vi "DaxsonicsGUI_3Pulsers.vi"(0 "Daxsonics VISA":refnum<visa-resource-name>="COM8", 5 "Daxsonics Name":T1, 11 "Uniform Gain":bool=TRUE) -> ()   [LabVIEW 2022 SP3]
doc: "This application VI allows the user to set the desired parameters in the Daxsonics BP2"
uses:
  -DaxSubroutines/Daxsonics_Pulsers.ctl
  PulserGlobals.vi
panel:
  in  "+12 dB Gain":bool
  in  "Element":u16(ring) items=["1", "2", "3", "4", "5"]
  in  "Delay Table (ns)":i32[][](array[numeric])=[[0, -1, -1, -1, -1], [-1, 0, -1, -1, -1], [-1, -1, 0, -1, -1], [-1, -1, -1, 0, -1], [-1, -1, -1, -1, 0]]
  in  "PRI":i32=500000
  in  "Trigger Rising (T)/Falling (F)":bool=TRUE
  in  "Trigger Ext(T)/Int(F)":bool
  in  "Freq (MHz)":u16(ring)=20 items=["50"=20, "45"=27, "40"=34, "35"=41, "30"=49, "25"=56, "20"=63, "15"=70]
  in  "Voltage (V)":u16(ring) items=["100"=100, "90"=90, "80"=80, "70"=70, "60"=60, "50"=50, "40"=40, "30"=30, "20"=20, "10"=10, "0"=0]
  in  "Gains (dB)":u16[](array[ring]) items=["64"=64, "60"=60, "52"=52, "48"=48, "44"=44, "40"=40, "36"=36, "32"=32, "28"=28, "24"=24, "20"=20, "16"=16]
  in  "Lock/Unlock":bool
  in  "ExitSendCmd":bool
  # "ONLY USED FOR 2021 NEW VERSION"
  # "Fixed 15.5 dB is start Gain"
  # "NUMTX = Rows\nColumn = Delays\n-1 means not used"
  # "Select xmit element (ie row)"
  # "Need to change COM port to these aliases based on daxsonics that is used\n\nDax2021 - newest Daxsonics from 2021\n\nor unites based on serial #\nDaxsonics_BP1 (faulty out of use)\nDaxsonics_BP2_A\nDaxsonics_BP2_B\n10ERS8 (this one is dead)"
  # "This is set up to pass one row"
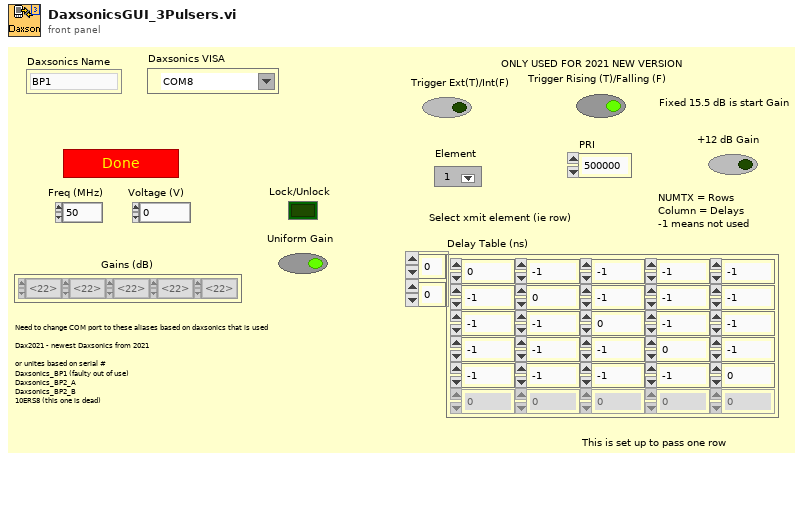
[diagram p1: front panel]
types:
  T1 = typedef "Daxsonics_Pulsers.ctl" = enum16{"BP1", "BP2_A", "BP2_B", "10ERS8", "New2021"}
  T2 = typedef "LVStringsAndValuesArrayTypeDef_U16.ctl" = cluster{"String":string, "Value":u16}[]
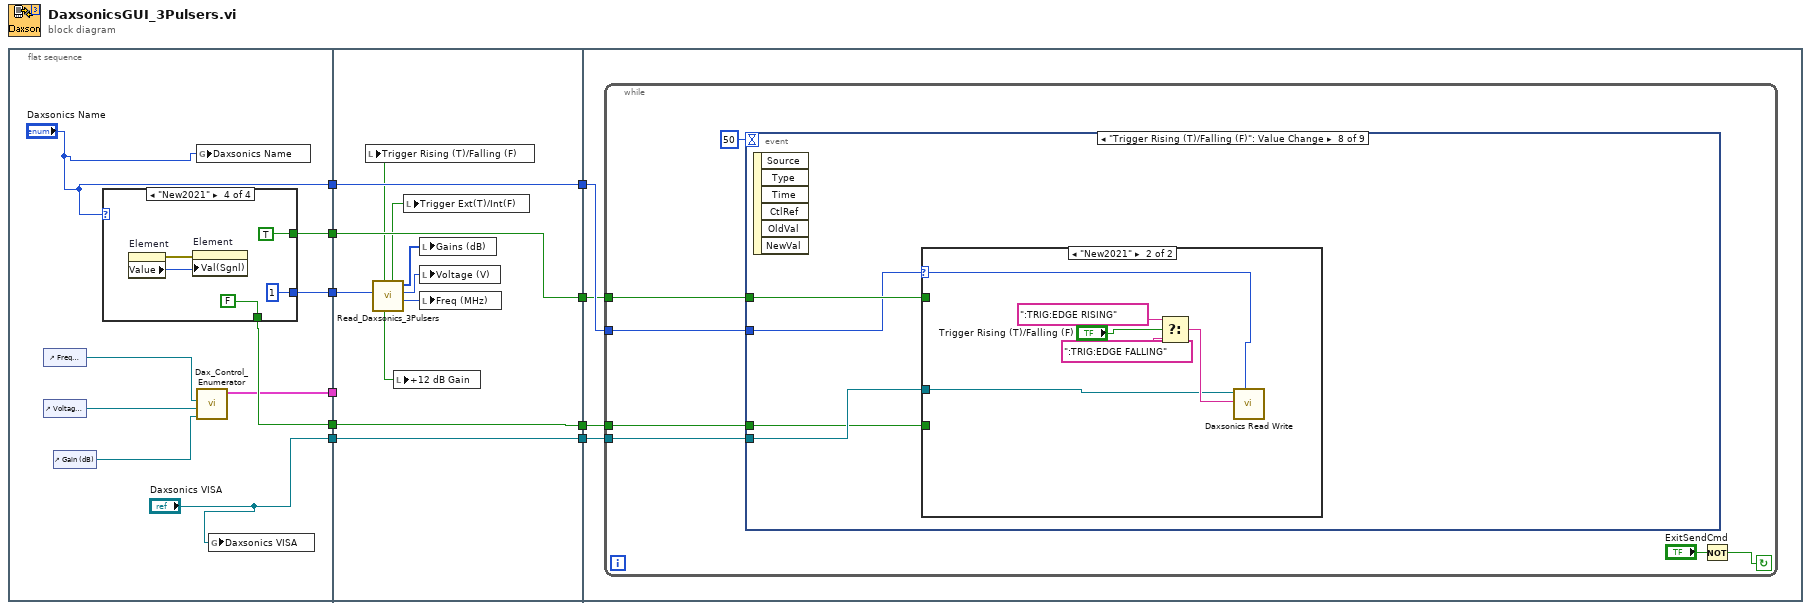
[diagram p0: block diagram]
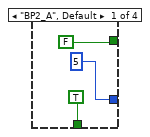
[diagram p2: hidden frame]
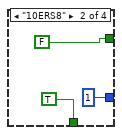
[diagram p3: hidden frame]
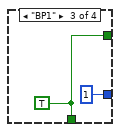
[diagram p4: hidden frame]
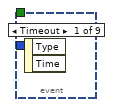
[diagram p5: hidden frame]
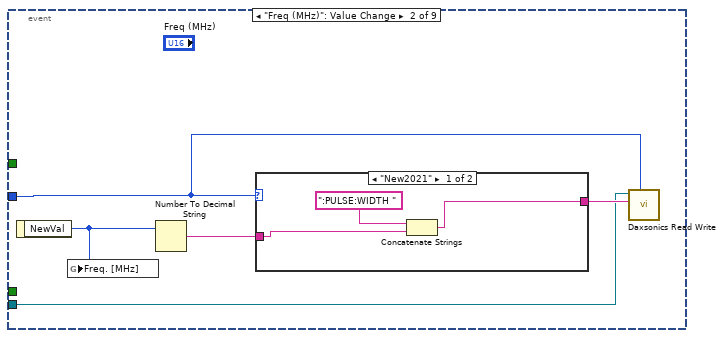
[diagram p6: hidden frame]
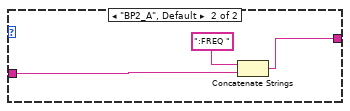
[diagram p7: hidden frame]
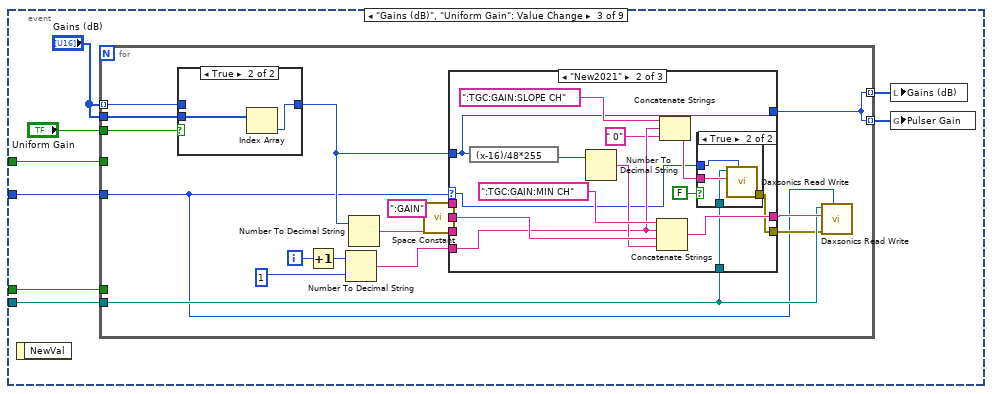
[diagram p8: hidden frame]
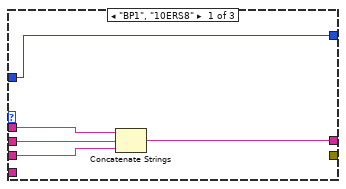
[diagram p9: hidden frame]
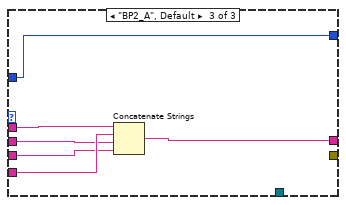
[diagram p11: hidden frame]
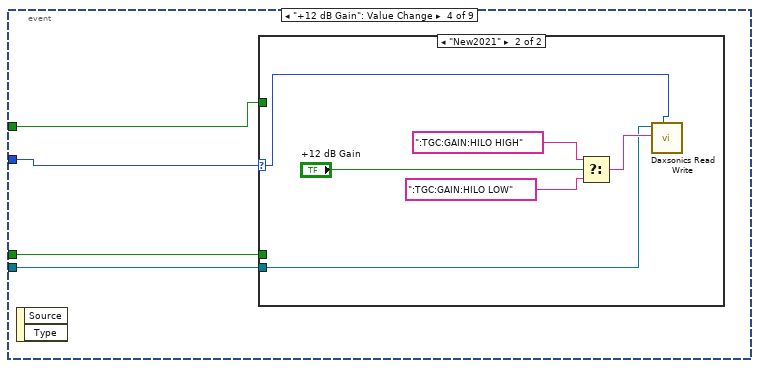
[diagram p13: hidden frame]
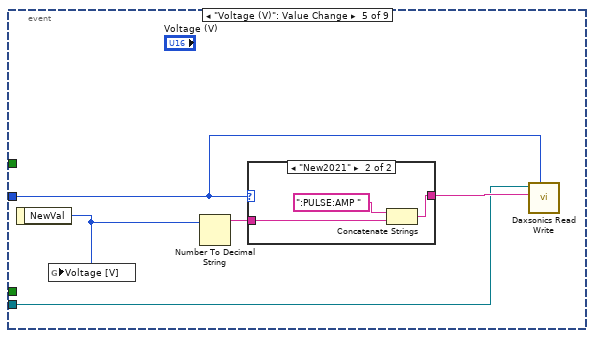
[diagram p15: hidden frame]
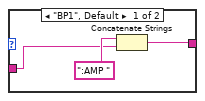
[diagram p16: hidden frame]
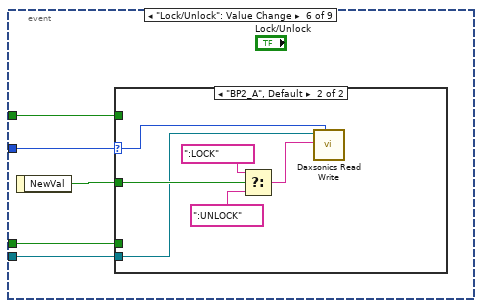
[diagram p17: hidden frame]
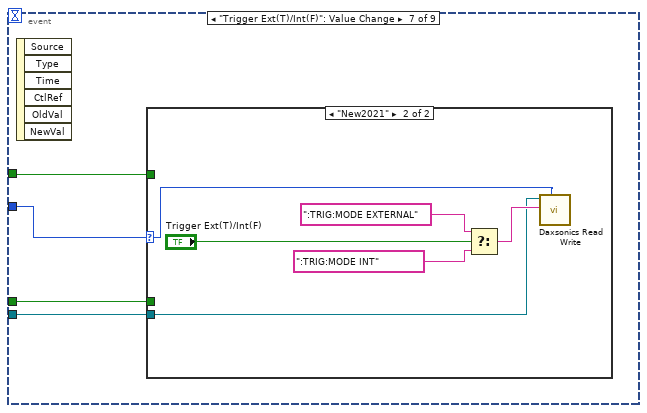
[diagram p19: hidden frame]
diagram:
  n1 = flat-sequence {
    tunnel: [w19] -> w9
    tunnel: ["Daxsonics Name"] -> w8
    tunnel: [w17] -> w5
    tunnel: [w14] -> w4
    tunnel: ["Daxsonics VISA"] -> w2
    tunnel: [w11] -> w1
    tunnel: [w33] -> w10
    tunnel: w9 -> [w40]
    tunnel: w8 -> [w39]
    tunnel: [w39] -> w7
    tunnel: [w38] -> w6
    tunnel: w5 -> [w38]
    tunnel: w4 -> [w37]
    tunnel: [w37] -> w3
    tunnel: w2 -> [w33]
    tunnel: w1 -> [_]
    tunnel: w10 -> [w47]
    tunnel: w7 -> [w46]
    tunnel: w6 -> [w45]
    tunnel: w3 -> [w44]
    frame #0 {
      n2 = control-ref of="Freq (MHz)"() -> (w18:refnum<vi>)
      n3 = control-ref of="Voltage (V)"() -> (w15:refnum<vi>)
      n4 = control-ref of="Gain (dB)"() -> (w16:refnum<vi>)
      n5 = case shown="\"New2021\"" "Daxsonics Name" {
        tunnel: [5 ("Num Channels") 1 ("Num Channels") 1 ("Num Channels") 1 ("Num Channels")] -> w19
        tunnel: [FALSE ("Enable Termination\nChar (T)") FALSE ("Enable Termination\nChar (T)") w26 TRUE ("Enable Termination\nChar (T)")] -> w17
        tunnel: [TRUE ("Enable Termination\nChar (T)") TRUE ("Enable Termination\nChar (T)") w26 FALSE ("Enable Termination\nChar (T)")] -> w14
        frame "BP2_A", Default {
        }
        frame "10ERS8" {
        }
        frame "BP1" {
          w26 = TRUE ("Enable Termination\nChar (T)")
        }
        frame "New2021" {
          n6 = property on="Element" class="Ring (strict)"() -> (error out=w29:errorcluster, "Value"=w28:u16)  [unwired: 2 in, 1 out]
          n7 = property on="Element" class="Ring (strict)"(error in=w29, "Val(Sgnl)"=w28) -> ()  [unwired: 1 in, 2 out]
        }
      }
      n8 = global write "PulserGlobals.vi" "Daxsonics Name"("Daxsonics Name") -> ()
      n9 = call "Dax_Control_Enumerator.vi"("Gain (dB) Ref"=w16, "Voltage (V) Ref"=w15, "Freq (MHz) Ref"=w18) -> ("Freq"=w11:T2)  [unwired: 6 in, 2 out]
      n10 = global write "PulserGlobals.vi" "Daxsonics VISA"("Daxsonics VISA") -> ()
    }
    frame #1 {
      n11 = call "Read_Daxsonics_3Pulsers.vi"("Num Channels"=w40) -> ("Freq (MHz)"=w43:u16, "Voltage (V)"=w42:u16, "Gains"=w41:u16[], "Trigger Ext(T)/Int(F)"=w35:bool, "HI(T)/LO(F) +12 dB"=w34:bool, "Trigger Rising (T)/Falling (F)"=w36:bool)  [unwired: 4 in, 1 out]
      n12 = local write "Trigger Rising (T)/Falling (F)"(w36) -> ()
      n13 = local write "+12 dB Gain"(w34) -> ()
      n14 = local write "Trigger Ext(T)/Int(F)"(w35) -> ()
      n15 = local write "Gains (dB)"(w41) -> ()
      n16 = local write "Voltage (V)"(w42) -> ()
      n17 = local write "Freq (MHz)"(w43) -> ()
    }
    frame #2 {
      n18 = while {
        tunnel: w47 -> [w51]
        tunnel: w46 -> [w50]
        tunnel: w45 -> [w49]
        tunnel: w44 -> [w48]
        stop <- w54 continue-if-true
        n19 = event shown="[7] \"Trigger Rising (T)/Falling (F)\": Value Change" {
          selector: _ -> [_ _ _ _ _ _ _ _ _]
          dyn-events: _ -> [_ _ _ _ _ _ _ _ _]
          timeout: 50 -> [_ _ _ _ _ _ _ _ _]
          tunnel: w51 -> [_ w56 w73 w123 w134 w146 w156 w166 w176]
          tunnel: w49 -> [_ _ w72 w124 _ w145 w157 w167 w175]
          tunnel: w50 -> [_ w55 w69 w125 w132 w144 w155 w164 w174]
          tunnel: w48 -> [_ _ w66 w122 _ w143 w154 w165 _]
          event Timeout {
            n20 = event-data() -> ()  [unwired: 3 out]
          }
          event "Freq (MHz)": Value Change {
            n21 = event-data() -> ("NewVal"=w58:u16)  [unwired: 1 out]
            n22 = global write "PulserGlobals.vi" "Freq. [MHz]"(w58) -> ()
            n23 = Number To Decimal String(number=w58) -> (decimal integer string=w59:string)  [unwired: 1 in]
            n24 = case shown="\"New2021\"" w55 {
              tunnel: w59 -> [w60 w64]
              tunnel: [w61 w63] -> w57
              frame "New2021" {
                n25 = Concatenate Strings(":PULSE:WIDTH " ("string"), w60) -> (w61:string)
              }
              frame "BP2_A", Default {
                n26 = Concatenate Strings(":FREQ " ("string"), w64) -> (w63:string)
              }
            }
            n27 = call "Daxsonics Read Write.vi"("Daxsonics Name"=w55, "write buffer"=w57, "VISA resource name"=w56) -> ()  [unwired: 6 in, 3 out]
          }
          event "Gains (dB)", "Uniform Gain": Value Change {
            n28 = event-data() -> ()  [unwired: 2 out]
            n29 = for {
              tunnel: "Gains (dB)" -> [w87] mode=indexing
              tunnel: w73 -> [w80]
              tunnel: [w75] -> w70 mode=indexing
              tunnel: w72 -> [_]
              tunnel: "Uniform Gain" -> [w86]
              tunnel: "Gains (dB)" -> [w85]
              tunnel: [w75] -> w71 mode=indexing
              tunnel: w69 -> [w74]
              tunnel: w66 -> [_]
              i -> [w89]
              n30 = case shown="True" w86 {
                tunnel: w87 -> [w119 _]
                tunnel: [w119 w120] -> w76
                tunnel: w85 -> [_ w121]
                frame False {
                }
                frame True {
                  n31 = Index Array(array=w121) -> (element=w120:u16)  [unwired: 1 in]
                }
              }
              n32 = Increment(x=w89) -> (x+1=w78:i32)
              n33 = Number To Decimal String(number=w78, width (-)=1) -> (decimal integer string=w88:string)
              n34 = Number To Decimal String(number=w76) -> (decimal integer string=w83:string)  [unwired: 1 in]
              n35 = call <vilib>:"Space Constant.vi"() -> ("String"=w81:string)
              n36 = case shown="\"New2021\"" w74 {
                selector: w74 -> [_ w95 _]
                tunnel: w88 -> [_ w103 w118]
                tunnel: ":GAIN" ("string") -> [w94 _ w117]
                tunnel: w83 -> [w93 _ w116]
                tunnel: [w92 w105 w114] -> w82
                tunnel: w81 -> [w91 w107 w115]
                tunnel: w76 -> [w90 w97 w113]
                tunnel: w80 -> [_ w100 _]
                tunnel: [_ w99 _] -> w79
                tunnel: [w90 w97 w113] -> w75
                frame "BP1", "10ERS8" {
                  n37 = Concatenate Strings(w94, w91, w93) -> (w92:string)
                }
                frame "New2021" {
                  n38 = expression code="(x-16)/48*255"(w97) -> (w98:u16)
                  n39 = Number To Decimal String(number=w98) -> (decimal integer string=w106:string)  [unwired: 1 in]
                  n40 = Concatenate Strings(":TGC:GAIN:MIN CH" ("string"), w103, w107, w106) -> (w105:string)
                  n41 = Concatenate Strings(":TGC:GAIN:SLOPE CH" ("string"), w103, " 0") -> (w101:string)
                  n42 = case shown="True" FALSE {
                    tunnel: w101 -> [_ w112]
                    tunnel: w100 -> [_ w111]
                    tunnel: [_ w110] -> w99
                    tunnel: w95 -> [_ w109]
                    frame False {
                    }
                    frame True {
                      n43 = call "Daxsonics Read Write.vi"("Daxsonics Name"=w109, "write buffer"=w112, "VISA resource name"=w111) -> ("error out"=w110:errorcluster)  [unwired: 6 in, 2 out]
                    }
                  }
                }
                frame "BP2_A", Default {
                  n44 = Concatenate Strings(w117, w118, w115, w116) -> (w114:string)
                }
              }
              n45 = call "Daxsonics Read Write.vi"("Daxsonics Name"=w74, "error IN"=w79, "write buffer"=w82, "VISA resource name"=w80) -> ()  [unwired: 5 in, 3 out]
            }
            n46 = local write "Gains (dB)"(w71) -> ()
            n47 = global write "PulserGlobals.vi" "Pulser Gain"(w70) -> ()
          }
          event "+12 dB Gain": Value Change {
            n48 = event-data() -> ()  [unwired: 3 out]
            n49 = case shown="\"New2021\"" w125 {
              selector: w125 -> [_ w126]
              tunnel: w124 -> [_ _]
              tunnel: w123 -> [_ w128]
              tunnel: w122 -> [_ _]
              frame "BP1", Default {
              }
              frame "New2021" {
                n50 = Select(t=":TGC:GAIN:HILO HIGH", s="+12 dB Gain", f=":TGC:GAIN:HILO LOW") -> (s? t:f=w131:string)
                n51 = call "Daxsonics Read Write.vi"("Daxsonics Name"=w126, "write buffer"=w131, "VISA resource name"=w128) -> ()  [unwired: 6 in, 3 out]
              }
            }
          }
          event "Voltage (V)": Value Change {
            n52 = event-data() -> ("NewVal"=w133:u16)  [unwired: 1 out]
            n53 = global write "PulserGlobals.vi" "Voltage [V]"(w133) -> ()
            n54 = Number To Decimal String(number=w133) -> (decimal integer string=w136:string)  [unwired: 1 in]
            n55 = case shown="\"New2021\"" w132 {
              tunnel: w136 -> [w137 w142]
              tunnel: [w138 w141] -> w135
              frame "BP1", Default {
                n56 = Concatenate Strings(":AMP " ("string"), w137) -> (w138:string)
              }
              frame "New2021" {
                n57 = Concatenate Strings(":PULSE:AMP " ("string"), w142) -> (w141:string)
              }
            }
            n58 = call "Daxsonics Read Write.vi"("Daxsonics Name"=w132, "write buffer"=w135, "VISA resource name"=w134) -> ()  [unwired: 6 in, 3 out]
          }
          event "Lock/Unlock": Value Change {
            n59 = event-data() -> ("NewVal"=w147:bool)  [unwired: 1 out]
            n60 = case shown="\"BP2_A\", Default" w144 {
              selector: w144 -> [_ w148]
              tunnel: w147 -> [_ w153]
              tunnel: w146 -> [_ w149]
              tunnel: w145 -> [_ _]
              tunnel: w143 -> [_ _]
              frame "New2021" {
              }
              frame "BP2_A", Default {
                n61 = Select(t=":LOCK", s=w153, f=":UNLOCK") -> (s? t:f=w150:string)
                n62 = call "Daxsonics Read Write.vi"("Daxsonics Name"=w148, "write buffer"=w150, "VISA resource name"=w149) -> ()  [unwired: 6 in, 3 out]
              }
            }
          }
          event "Trigger Ext(T)/Int(F)": Value Change {
            n63 = event-data() -> ()  [unwired: 7 out]
            n64 = case shown="\"New2021\"" w155 {
              selector: w155 -> [_ w158]
              tunnel: w157 -> [_ _]
              tunnel: w156 -> [_ w159]
              tunnel: w154 -> [_ _]
              frame "BP1", Default {
              }
              frame "New2021" {
                n65 = Select(t=":TRIG:MODE EXTERNAL", s="Trigger Ext(T)/Int(F)", f=":TRIG:MODE INT") -> (s? t:f=w163:string)
                n66 = call "Daxsonics Read Write.vi"("Daxsonics Name"=w158, "write buffer"=w163, "VISA resource name"=w159) -> ()  [unwired: 6 in, 3 out]
              }
            }
          }
          event "Trigger Rising (T)/Falling (F)": Value Change {
            n67 = event-data() -> ()  [unwired: 7 out]
            n68 = case shown="\"New2021\"" w164 {
              selector: w164 -> [_ w168]
              tunnel: w167 -> [_ _]
              tunnel: w166 -> [_ w172]
              tunnel: w165 -> [_ _]
              frame "BP1", Default {
              }
              frame "New2021" {
                n69 = Select(t=":TRIG:EDGE RISING", s="Trigger Rising (T)/Falling (F)", f=":TRIG:EDGE FALLING") -> (s? t:f=w173:string)
                n70 = call "Daxsonics Read Write.vi"("Daxsonics Name"=w168, "write buffer"=w173, "VISA resource name"=w172) -> ()  [unwired: 6 in, 3 out]
              }
            }
          }
          event "Delay Table (ns)", "Element", "PRI": Value Change {
            n71 = event-data() -> ()  [unwired: 7 out]
            n72 = case shown="\"New2021\"" w174 {
              selector: w174 -> [_ w177]
              tunnel: w176 -> [_ w183]
              tunnel: w175 -> [_ _]
              frame "BP1", Default {
              }
              frame "New2021" {
                n73 = case shown="True" TRUE {
                  tunnel: "Delay Table (ns)" -> [w184 w188]
                  tunnel: "Element" -> [_ w187]
                  tunnel: [w184 w185] -> w181
                  frame False {
                  }
                  frame True {
                    n74 = Index Array(array=w188, index (row)=w187) -> (element=w186:i32[])  [unwired: 1 in]
                    n75 = Build Array(w186) -> (w185:i32[][])
                  }
                }
                n76 = call "DelayTableLoad.vi"("Daxsonics Name"=w177, "PRI (ns)"="PRI", "Delay Table (ns)"=w181, "VISA Refnum in"=w183) -> ()  [unwired: 8 in]
              }
            }
          }
        }
        n77 = Not(x="ExitSendCmd") -> (.not. x?=w54:bool)
      }
    }
  }
